vi "Spring Model.vi"(4 "Vy":dbl, 6 "Vx":dbl, 7 "Parameters":T1={"Spring Stiffness"=0.1, "Deadzone Radius"=0.1, "Damping Co-efficient"=0.08}, 8 "Current Y":dbl=17.7178955078125, 9 "Current X":dbl=85.089111328125, 10 "Target Y":dbl=-128.10971069335938, 11 "Target X":dbl=-76.65448760986328) -> (1 "F_vector":cdb[](array[numeric]))   [LabVIEW 2017, in "myPAM.lvlib"]
uses:
  myPAM.lvlib
  <vilib>/imath/engines/lvmath2/RunTimeEngine/ArithmeticOperatorToken/NIMS_ArithmeticOperator_minus.vi
  <instcachedir>/0/NIMS_ArithmeticOperator_minus_0AD0C6F3574E48218C82EC0DAEF38AC8.lvgen/NIMS_ArithmeticOperator_minus_0AD0C6F3574E48218C82EC0DAEF38AC8_003.vi
  <vilib>/imathl/engines/lvmath/Functions/Error Handling/Create Error.vi
  <vilib>/imath/engines/lvmath2/RunTimeEngine/BuiltInFunctions/abs/NIMS_abs(signed).vi
  <instcachedir>/0/NIMS_abs(signed)_C4FCB8E6058B49B797C7C8D53CA5F6EC.lvgen/NIMS_abs(signed)_C4FCB8E6058B49B797C7C8D53CA5F6EC_001.vi
  <vilib>/imath/engines/lvmath2/RunTimeEngine/IndexRead/NIMS V(S).vi
  <instcachedir>/0/NIMS V(S)_0488751826AF41519A22953C041130DC.lvgen/NIMS V(S)_0488751826AF41519A22953C041130DC_003.vi
  <vilib>/imath/engines/lvmath2/RunTimeEngine/BuiltInFunctions/min/1 input/NIMS_min(RV).vi
  <instcachedir>/0/NIMS_min(RV)_EE2DD3E2888846108C5160A664B67832.lvgen/NIMS_min(RV)_EE2DD3E2888846108C5160A664B67832_000.vi
  <instcachedir>/0/NIMS V(S)_0488751826AF41519A22953C041130DC.lvgen/NIMS V(S)_0488751826AF41519A22953C041130DC_000.vi
  <vilib>/imath/engines/lvmath2/RunTimeEngine/IndexReplace/NIMS V(S)=S.vi
  <instcachedir>/0/NIMS V(S)=S_3F4D177D41884A9C969E5FA0B22E4B28.lvgen/NIMS V(S)=S_3F4D177D41884A9C969E5FA0B22E4B28_000.vi
  <vilib>/imath/engines/lvmath2/RunTimeEngine/ArithmeticOperatorToken/NIMS_ArithmeticOperator_rightdiv.vi
  <instcachedir>/0/NIMS_ArithmeticOperator_rightdiv_EFA95513F40C4B3084B27C9DE6D5A167.lvgen/NIMS_ArithmeticOperator_rightdiv_EFA95513F40C4B3084B27C9DE6D5A167_000.vi
  <vilib>/imath/engines/lvmath2/RunTimeEngine/BuiltInFunctions/max/2 inputs/NIMS_max(RG,RG)-no size check.vi
  <instcachedir>/0/NIMS_max(RG,RG)-no size check_F871939977644B7683C1350DCCAD7557.lvgen/NIMS_max(RG,RG)-no size check_F871939977644B7683C1350DCCAD7557_001.vi
  <vilib>/imath/engines/lvmath2/RunTimeEngine/BuiltInFunctions/min/2 inputs/NIMS_min(RG,RG)-no size check.vi
  <instcachedir>/0/NIMS_min(RG,RG)-no size check_7F67BAB91AFC452D9517D2EA1C8F5F88.lvgen/NIMS_min(RG,RG)-no size check_7F67BAB91AFC452D9517D2EA1C8F5F88_001.vi
  <vilib>/imath/engines/lvmath2/RunTimeEngine/ArithmeticOperatorToken/NIMS_ArithmeticOperator_times.vi
  <instcachedir>/0/NIMS_ArithmeticOperator_times_9BECD6C28351466A83A029AF2762CD58.lvgen/NIMS_ArithmeticOperator_times_9BECD6C28351466A83A029AF2762CD58_000.vi
  <vilib>/imath/engines/lvmath2/RunTimeEngine/ArithmeticOperatorToken/NIMS_ArithmeticOperator_plus.vi
  <instcachedir>/0/NIMS_ArithmeticOperator_plus_9255C7DA94A9479C92F91DC2DA9A664F.lvgen/NIMS_ArithmeticOperator_plus_9255C7DA94A9479C92F91DC2DA9A664F_004.vi
  <vilib>/imath/engines/lvmath2/RunTimeEngine/ErrorHandling/NIMS_Create Error From Enums.vi
  <vilib>/imath/engines/lvmath2/RunTimeEngine/NodeEndStatement/NIMS_NodeEndStatement_Output.vi
  <instcachedir>/0/NIMS_NodeEndStatement_Output_53EC0D466D134D7ABD903AC30B43404B.lvgen/NIMS_NodeEndStatement_Output_53EC0D466D134D7ABD903AC30B43404B_010.vi
  <instcachedir>/0/NIMS_NodeEndStatement_Output_53EC0D466D134D7ABD903AC30B43404B.lvgen/NIMS_NodeEndStatement_Output_53EC0D466D134D7ABD903AC30B43404B_005.vi
  <vilib>/imath/engines/lvmath2/RunTimeEngine/ErrorHandling/NIMS_Finalize Error.vi
panel:
  in  "Vmax":dbl(slide) scale=50.0..500.0
  out "satu":bool[](array[boolean])
  out "F_re":dbl[](array[numeric])
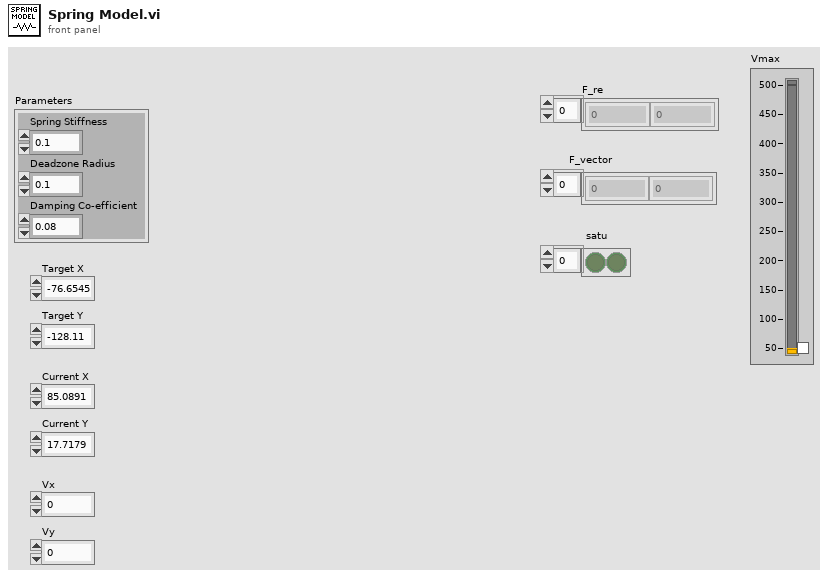
[diagram p1: front panel]
types:
  T1 = cluster{"Spring Stiffness":dbl, "Deadzone Radius":dbl, "Damping Co-efficient":dbl}
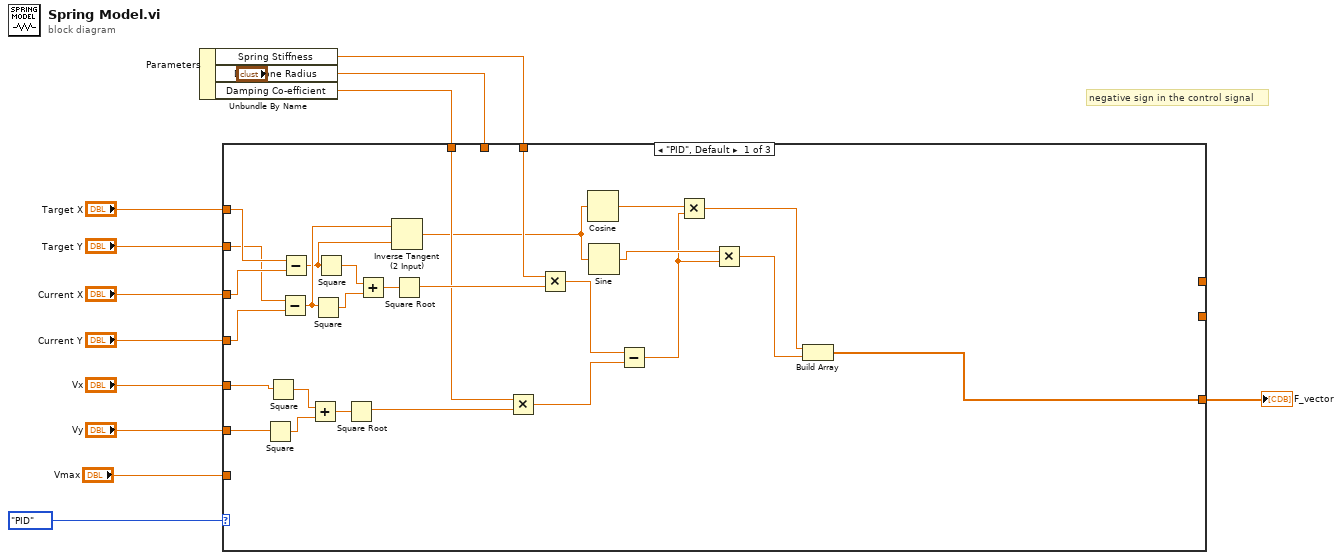
[diagram p0: block diagram]
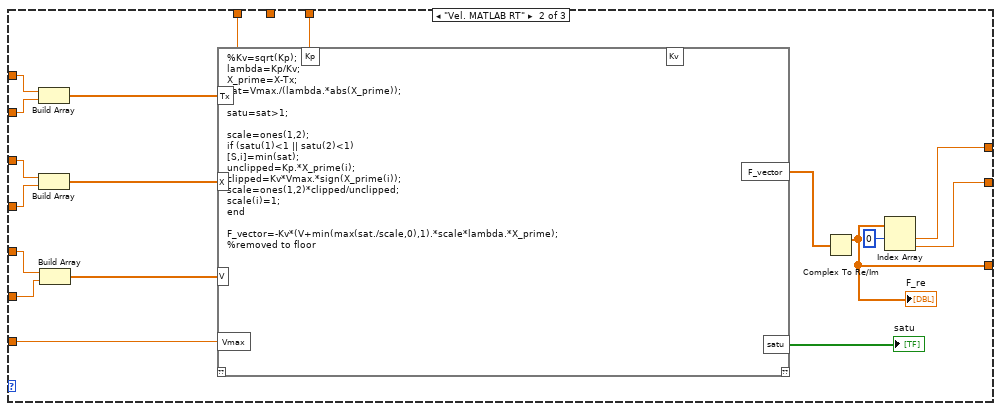
[diagram p2: hidden frame]
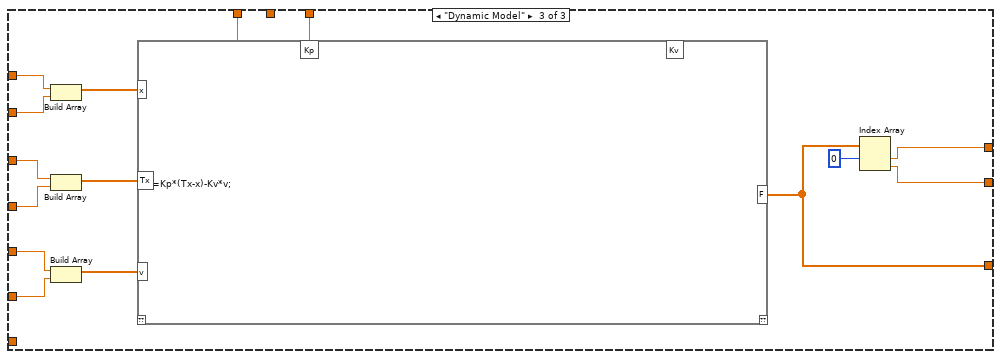
[diagram p3: hidden frame]
diagram:
  # "negative sign in the control signal"
  n1 = Unbundle By Name("Parameters") -> ("Spring Stiffness"=w4:dbl, "Deadzone Radius"=w12:dbl, "Damping Co-efficient"=w5:dbl)
  n2 = case shown="\"PID\", Default" enum16{"Vel. MATLAB RT", "Dynamic Model", "PID"}."PID" {
    tunnel: w12 -> [_ _ _]
    tunnel: "Target X" -> [w40 w58 w341]
    tunnel: "Current X" -> [w39 w55 w339]
    tunnel: "Target Y" -> [w38 w57 w340]
    tunnel: "Current Y" -> [w37 w54 w338]
    tunnel: "Vx" -> [w28 w52 w337]
    tunnel: "Vy" -> [w27 w51 w336]
    tunnel: "Vmax" -> [_ w47 _]
    tunnel: [_ w45 w329] -> _
    tunnel: [_ w44 w328] -> _
    tunnel: w5 -> [w23 w48 w331]
    tunnel: w4 -> [w26 w49 w332]
    tunnel: [w20 w42 w327] -> w2
    frame "PID", Default {
      n3 = Square(x=w27) -> (x^2=w30:dbl)
      n4 = Square(x=w28) -> (x^2=w29:dbl)
      n5 = Subtract(x=w38, y=w37) -> (x-y=w33:dbl)
      n6 = Subtract(x=w40, y=w39) -> (x-y=w32:dbl)
      n7 = Add(x=w29, y=w30) -> (x+y=w31:dbl)
      n8 = Square(x=w33) -> (x^2=w36:dbl)
      n9 = Square(x=w32) -> (x^2=w35:dbl)
      n10 = Square Root(x=w31) -> (sqrt(x)=w22:dbl)
      n11 = Add(x=w35, y=w36) -> (x+y=w34:dbl)
      n12 = Inverse Tangent (2 Input)(1:w32, 2:w33) -> (0:w19:dbl)
      n13 = Square Root(x=w34) -> (sqrt(x)=w25:dbl)
      n14 = Multiply(x=w23, y=w22) -> (x*y=w21:dbl)
      n15 = Multiply(x=w26, y=w25) -> (x*y=w24:dbl)
      n16 = Cosine(x=w19) -> (cos(x)=w18:dbl)
      n17 = Sine(x=w19) -> (sin(x)=w17:dbl)
      n18 = Subtract(x=w24, y=w21) -> (x-y=w16:dbl)
      n19 = Multiply(x=w18, y=w16) -> (x*y=w15:dbl)
      n20 = Multiply(x=w17, y=w16) -> (x*y=w14:dbl)
      n21 = Build Array(w15, w14) -> (w20:dbl[])
    }
    frame "Vel. MATLAB RT" {
      n22 = Build Array(w58, w57) -> (w56:dbl[])
      n23 = Build Array(w55, w54) -> (w53:dbl[])
      n24 = Build Array(w52, w51) -> (w50:dbl[])
      n25 = mathscript code="%Kv=sqrt(Kp);\nlambda=Kp/Kv;\nX_prime=X-Tx;\nsat=Vmax./(lambda.*abs(X_prime));\n\nsatu=sat>1;\n\nscale=ones(1,2);\nif (satu(1)<1 || satu(2)<1)\n[S,i]=min(sat);\nunclipped=Kp.*X_prime(i);\nclipped=Kv*Vmax.*sign(X_prime(i));\nscale=ones(1,2)*clipped/unclipped;\nscale(i)=1;\nend\n\nF_vector=-Kv*(V+min(max(sat./scale,0),1).*scale*lambda.*X_prime);\n%removed to floor"("Tx"=w56, "X"=w53, "V"=w50, "Vmax"=w47, "Kp"=w49, "Kv"=w48) -> ("F_vector"=w46:dbl[], "satu"=→"satu":bool[])  [unwired: 1 in, 1 out]
      n26 = Complex To Re/Im(x + iy=w46) -> (x=w42:dbl[])  [unwired: 1 out]
      "F_re" <- w42
      n27 = Index Array(array=w42, index #1=0 ("index")) -> (element #1=w45:dbl, element #2=w44:dbl)  [unwired: 1 in]
    }
    frame "Dynamic Model" {
      n28 = Build Array(w341, w340) -> (w335:dbl[])
      n29 = Build Array(w339, w338) -> (w334:dbl[])
      n30 = Build Array(w337, w336) -> (w333:dbl[])
      n31 = mathscript code="F=Kp*(Tx-x)-Kv*v;"("x"=w335, "Tx"=w334, "v"=w333, "Kp"=w332, "Kv"=w331) -> ("F"=w327:dbl[])  [unwired: 1 in, 1 out]
      n32 = Index Array(array=w327, index #1=0 ("index")) -> (element #1=w329:dbl, element #2=w328:dbl)  [unwired: 1 in]
    }
  }
  "F_vector" <- w2
